vi "MIN MAX Without using Comparison.vi"(10 "NUM 2":dbl, 11 "NUM 1":dbl) -> (2 "MIN":dbl, 3 "Max":dbl)   [LabVIEW 2020]
doc: "This VI will be giving out Minimum and Maximum from given two numbers without using the comparison operator."
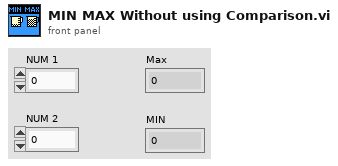
[diagram p1: front panel]
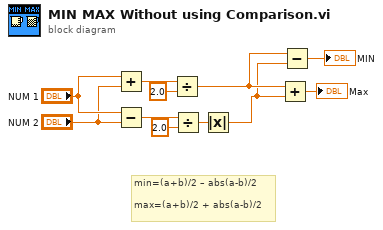
[diagram p0: block diagram]
diagram:
  # "min=(a+b)/2 – abs(a-b)/2\n\nmax=(a+b)/2 + abs(a-b)/2"
  n1 = Add(x="NUM 1", y="NUM 2") -> (x+y=w11:dbl)
  n2 = Subtract(x="NUM 1", y="NUM 2") -> (x-y=w7:dbl)
  n3 = Divide(x=w11, y=2.0) -> (x/y=w3:dbl)
  n4 = Divide(x=w7, y=2.0) -> (x/y=w5:dbl)
  n5 = Absolute Value(x=w5) -> (abs(x)=w2:dbl)
  n6 = Add(x=w3, y=w2) -> (x+y=→"Max":dbl)
  n7 = Subtract(x=w3, y=w2) -> (x-y=→"MIN":dbl)
